vi "Create.vi"(0 "Type":string, 7 "Target":string) -> (8 "Timeout":refnum<class "Timeout.lvclass">)   [LabVIEW 2020, in "Timeout.lvclass"]
uses:
  Timeout.lvclass
  Typedefs/Tosca-Event Type.ctl
  Timeout.lvclass/Timeout.ctl
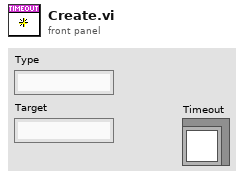
[diagram p1: front panel]
types:
  T1 = typedef "Tosca-Event Type.ctl" = enum16{"Normal", "CS+", "CS-"}
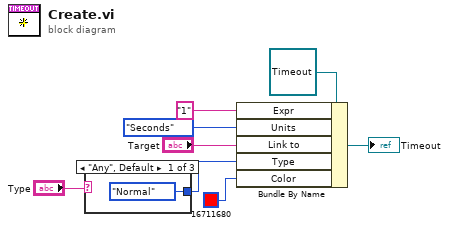
[diagram p0: block diagram]
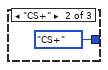
[diagram p2: hidden frame]
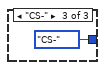
[diagram p3: hidden frame]
diagram:
  n1 = case shown="\"Any\", Default" "Type" {
    tunnel: [Tosca-Event_Type."Normal" ("Serialized.Type") Tosca-Event_Type."CS+" ("Serialized.Type") Tosca-Event_Type."CS-" ("Serialized.Type")] -> w2
    frame "Any", Default {
    }
    frame "CS+" {
    }
    frame "CS-" {
    }
  }
  n2 = Bundle By Name(cluster=refnum<class "Timeout.lvclass"> refnum ("Timeout"), "Expr"="1" ("Serialized.Expr"), "Units"=enum16{"Reps", "Seconds"}."Seconds" ("Serialized.Units"), "Link to"="Target", "Type"=w2, "Color"=u32 16711680) -> (→"Timeout":refnum<class "Timeout.lvclass">)
